vi "Create New Service.vi"(8 "error in (no error)":errorcluster, 10 "Name":string, 11 "Service in":refnum<class "Service.lvclass">) -> (0 "error out":errorcluster, 3 "Service out":refnum<class "Service.lvclass">)   [LabVIEW 2024, in "Ramses Framework.lvlib" / "Service.lvclass"]
uses:
  Service.lvclass
  Service.lvclass/Service.ctl
  Communications/Server/Base Server/Server.lvclass
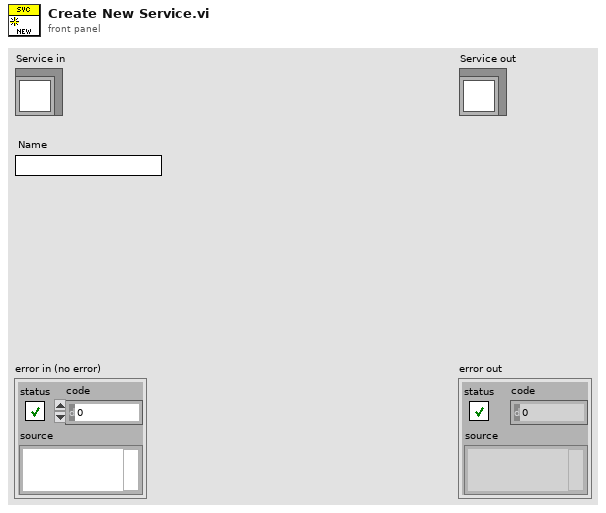
[diagram p1: front panel]
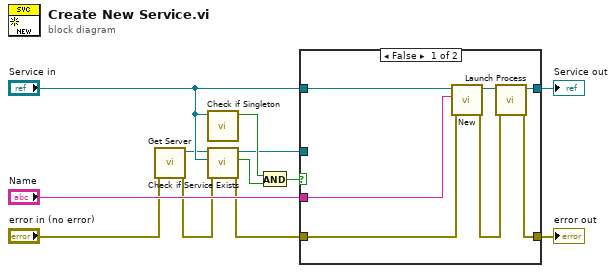
[diagram p0: block diagram]
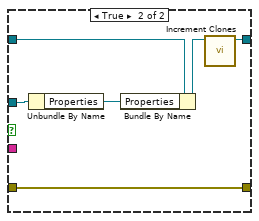
[diagram p2: hidden frame]
diagram:
  n1 = call "Get Server.vi"("error in (no error)"="error in (no error)") -> ("error out"=w1:errorcluster, "Server out"=w3:refnum<class "Server.lvclass">)  [unwired: 9 in]
  n2 = call-dynamic "Check if Singleton.vi"("Service in"="Service in") -> ("Singleton?"=w5:bool)  [unwired: 9 in, 1 out]
  n3 = call-dynamic "Check if Service Exists.vi"("error in (no error)"=w1, "Service in"="Service in", "Server in"=w3) -> ("error out"=w9:errorcluster, "Service Exists"=w8:bool, "Service out"=w4:refnum<class "Service.lvclass">)  [unwired: 6 in]
  n4 = And(x=w5, y=w8) -> (x .and. y?=w7:bool)
  n5 = case shown="False" w7 {
    tunnel: "Name" -> [w19 _]
    tunnel: w9 -> [w18 w25]
    tunnel: "Service in" -> [w17 w23]
    tunnel: [w15 w24] -> w11
    tunnel: [w13 w25] -> w10
    tunnel: w4 -> [_ w21]
    frame False {
      n6 = call-dynamic "New.vi"("error in (no error)"=w18, "Name"=w19, "Service in"=w17) -> ("error out"=w14:errorcluster, "Service out"=w16:refnum<class "Service.lvclass">)  [unwired: 7 in]
      n7 = call "Launch Process.vi"("error in (no error)"=w14, "Service in"=w16) -> ("error out"=w13:errorcluster, "Service out"=w15:refnum<class "Service.lvclass">)  [unwired: 8 in]
    }
    frame True {
      n8 = Unbundle By Name(w21) -> ("Properties"=w20:refnum<data-value>)
      n9 = Bundle By Name(cluster=w23, "Properties"=w20) -> (w22:refnum<class "Service.lvclass">)
      n10 = call "Increment Clones.vi"("Service in"=w22) -> ("Service out"=w24:refnum<class "Service.lvclass">)  [unwired: 9 in, 1 out]
    }
  }
  "error out" <- w10
  "Service out" <- w11
